vi "SV Stationary Loudness.vi"   [LabVIEW 2017, in "SoundVib_SoundQuality.lvlib"]
doc: "Computes stationary loudness from the sound pressure signal waveform or the 1/3-octave band spectrum calculated over the frequency range 25 Hz to 12.5 kHz. Wire data to the <B>sound pressure signal [Pa]</B> input to determine the polymorphic instance to use or manually select the instance."
uses:
  <vilib>/addons/Sound and Vibration/svt_Sound Quality/SoundVib_SoundQuality.lvlib
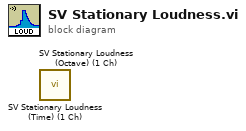
[diagram p0: block diagram]
diagram:
  n1 = call <vilib>:"SV Stationary Loudness (Time) (1 Ch).vi"() -> ()  [unwired: 11 in, 5 out]
  n2 = call <vilib>:"SV Stationary Loudness (Octave) (1 Ch).vi"() -> ()  [unwired: 11 in, 5 out]
